vi "Next Instance Number.vi"(8 "error in (no error)":errorcluster, 10 "Module Type":T2, 11 "Operation":T1) -> (0 "error out":errorcluster, 3 "Instance Number":i32)   [LabVIEW 2018, in "Drag and Drop.lvlib"]
uses:
  Drag and Drop.lvlib
  Module Type Enum.ctl
  Module Instance Number Operation Enum.ctl
panel:
  out "Instance Numbers":i32[](array[numeric])
  out "Strings []":string[](array[string])
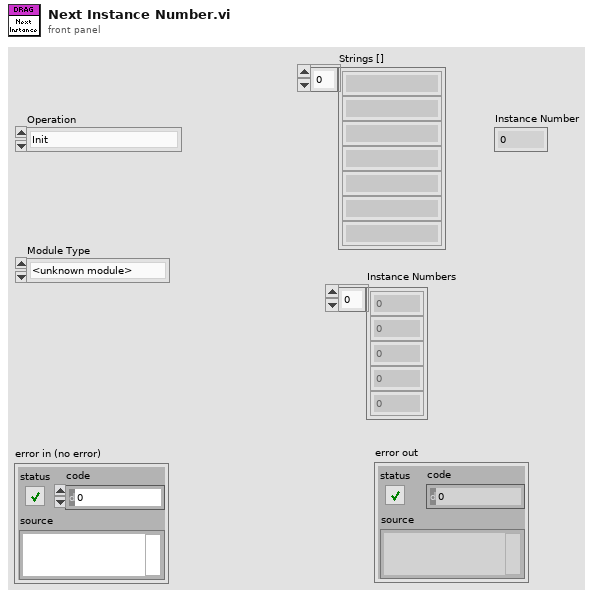
[diagram p1: front panel]
types:
  T1 = typedef "Module Instance Number Operation Enum.ctl" = enum16{"Init", "Next Instance Number"}
  T2 = typedef "Drag and Drop.lvlib/Module Type Enum.ctl" = enum16{"<unknown module>", "Feed", "TT", "PT", "Scale", "Flow", "Pump", "U3", "TCU", "DO", "PR", "OPC"}
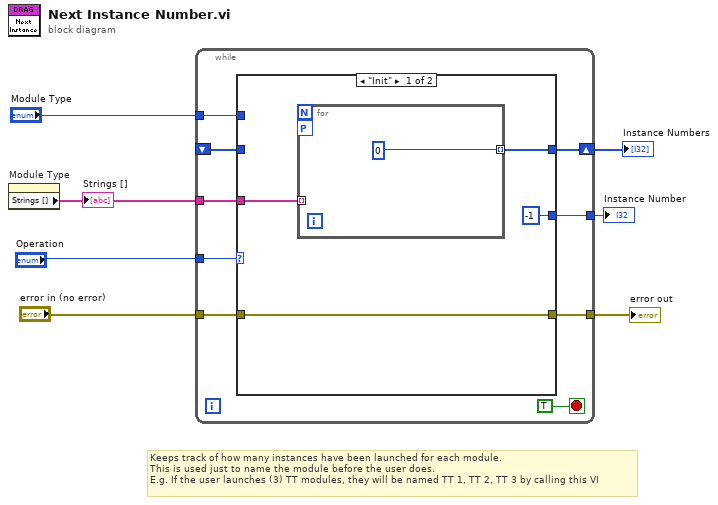
[diagram p0: block diagram]
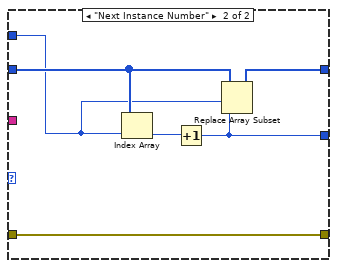
[diagram p2: hidden frame]
diagram:
  # "Keeps track of how many instances have been launched for each module.\nThis is used just to name the module before the user does.\nE.g. If the user launches (3) TT modules, they will be named TT 1, TT 2, TT 3 by calling this VI"
  n1 = property on="Module Type" class="Enum (strict)"() -> ("Strings []"=w4:string[])  [unwired: 2 in, 2 out]
  "Strings []" <- w4
  n2 = while {
    tunnel: "Operation" -> [w16]
    shift-right: [w12] -> w3
    shift-left: _ -> [w11]
    tunnel: [w15] -> w6
    tunnel: "error in (no error)" -> [w14]
    tunnel: w4 -> [w13]
    tunnel: "Module Type" -> [w10]
    tunnel: [w9] -> w1
    stop <- TRUE stop-if-true
    n3 = case shown="\"Init\"" w16 {
      tunnel: [w20 w22] -> w15
      tunnel: w14 -> [w20 w22]
      tunnel: w13 -> [w19 _]
      tunnel: [w18 w26] -> w12
      tunnel: w11 -> [_ w27]
      tunnel: w10 -> [_ w25]
      tunnel: [-1 w23] -> w9
      frame "Init" {
        n4 = for {
          tunnel: w19 -> [_] mode=indexing
          tunnel: [0] -> w18 mode=indexing
          workers-P: _ -> [_]
        }
      }
      frame "Next Instance Number" {
        n5 = Index Array(array=w27, index=w25) -> (element=w24:i32)
        n6 = Increment(x=w24) -> (x+1=w23:i32)
        n7 = Replace Array Subset(array=w27, new element=w23, index=w25) -> (w26:i32[])
      }
    }
  }
  "error out" <- w6
  "Instance Numbers" <- w3
  "Instance Number" <- w1
